vi "Sleep Test.vi"() -> ()   [LabVIEW 2013]
uses:
  Source/Controls/Public/C Enums/clockid_t.ctl
  Source/VIs/Public/Time/Get Clock Time (timespec).vi
  Source/VIs/Public/Time/Nanosleep Absolute (timespec).vi
  Source/Linux RT Utilities.lvlib
panel:
  out "Loop 1":i32
  out "Loop 2":i32
  in  "stop":bool
  in  "Period (ns)":i64=1000000 format="%#.3p"
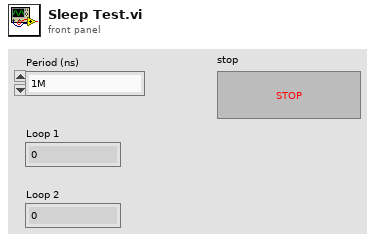
[diagram p1: front panel]
types:
  T1 = typedef "Linux RT Utilities.lvlib/clockid_t.ctl" = enum16{"Realtime", "Monotonic"}
  T2 = typedef "Linux RT Utilities.lvlib/timespec_64.ctl" = cluster{"sec":u64, "nsec":u64}
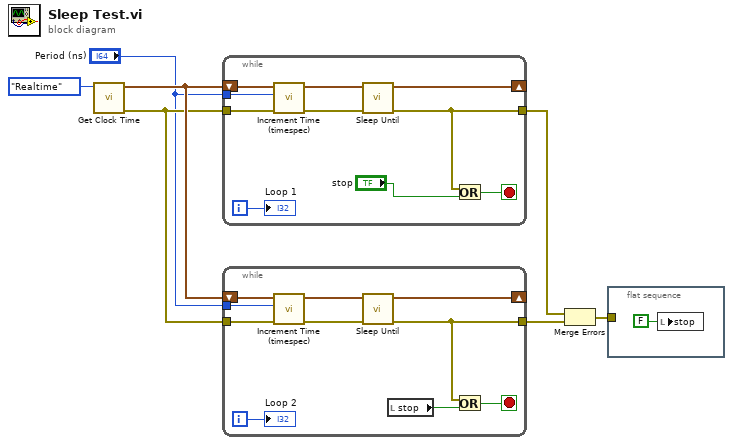
[diagram p0: block diagram]
diagram:
  n1 = call-poly "Get Clock Time.vi"("clock id (realtime)"=clockid_t."Realtime" ("clock id (monotonic)")) -> ("error out"=w3:errorcluster, "timespec"=w4:T2)  [unwired: 9 in]
  n2 = while {
    tunnel: w3 -> [w16]
    shift-right: [w9] -> _
    shift-left: w4 -> [w17]
    tunnel: "Period (ns)" -> [w15]
    tunnel: [w11] -> w1
    i -> [w12]
    stop <- w13 stop-if-true
    n3 = call "Increment Time (timespec).vi"("error in (no error)"=w16, "nanoseconds to add"=w15, "timespec in"=w17) -> ("error out"=w14:errorcluster, "timespec out"=w10:T2)  [unwired: 7 in]
    n4 = call-poly "Sleep Until.vi"("error in (no error)"=w14, "sleep until (timespec)"=w10) -> ("error out"=w11:errorcluster, "current time (timspec)"=w9:T2)  [unwired: 8 in]
    n5 = Or(x=w11, y="stop") -> (x .or. y?=w13:bool)
    "Loop 1" <- w12
  }
  n6 = while {
    tunnel: w3 -> [w26]
    shift-right: [w18] -> _
    shift-left: w4 -> [w27]
    tunnel: "Period (ns)" -> [w25]
    tunnel: [w20] -> w7
    i -> [w22]
    stop <- w23 stop-if-true
    n7 = call "Increment Time (timespec).vi"("error in (no error)"=w26, "nanoseconds to add"=w25, "timespec in"=w27) -> ("error out"=w24:errorcluster, "timespec out"=w19:T2)  [unwired: 7 in]
    n8 = call-poly "Sleep Until.vi"("error in (no error)"=w24, "sleep until (timespec)"=w19) -> ("error out"=w20:errorcluster, "current time (timspec)"=w18:T2)  [unwired: 8 in]
    n9 = local read "stop"() -> (w21:bool)
    n10 = Or(x=w20, y=w21) -> (x .or. y?=w23:bool)
    "Loop 2" <- w22
  }
  n11 = Merge Errors(w1, w7) -> (w6:errorcluster)
  n12 = flat-sequence {
    tunnel: w6 -> [_]
    frame #0 {
      n13 = local write "stop"(FALSE ("stop")) -> ()
    }
  }
